vi "Configure SPI Source.vi"(7 "Source Type (0: Clock Source)":i32(ring) items=["Clock Source", "Data Source", "Frame Source", "MISO Source", "MOSI Source"], 8 "error in (no error)":errorcluster, 9 "SPI Source (0: Channel 1)":i32(ring) items=["Channel 1", "Channel 2", "Channel 3", "Channel 4", "Function 1", "Function 2", "Function 3", "Function 4", "Memory 1", "Memory 2", "Memory 3", "Memory 4", "Digital 0", "Digital 1", "Digital 2", "Digital 3", "Digital 4", "Digital 5", "Digital 6", "Digital 7", "Digital 8", "Digital 9", "Digital 10", "Digital 11", "Digital 12", "Digital 13", "Digital 14", "Digital 15"], 10 "Channel (1: Serial Bus 1)":i32(ring)=1 items=["Serial Bus 1"=1, "Serial Bus 2"=2, "Serial Bus 3"=3, "Serial Bus 4"=4], 11 "VISA resource name":refnum<visa-resource-name>) -> (0 "error out":errorcluster, 3 "VISA resource name out":refnum<visa-resource-name>)   [LabVIEW 2020, in "Agilent 90000 Series.lvlib"]
doc: "Configures the source for SPI serial bus."
uses:
  Agilent 90000 Series.lvlib
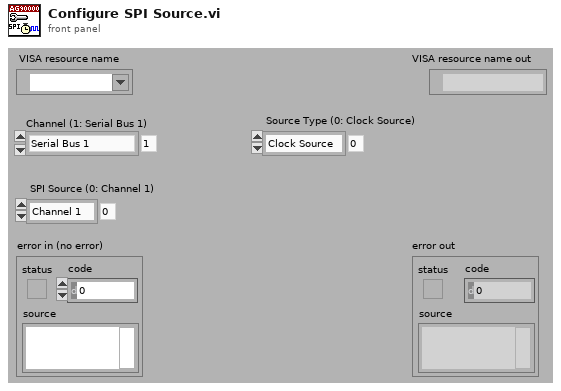
[diagram p1: front panel]
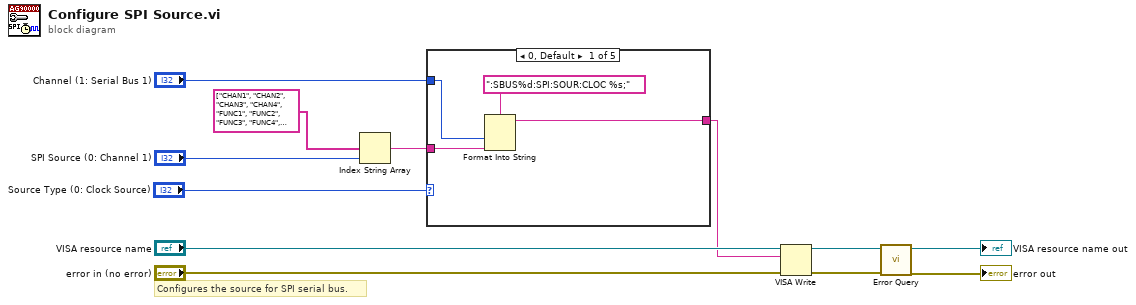
[diagram p0: block diagram]
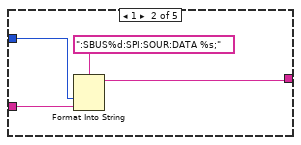
[diagram p2: hidden frame]
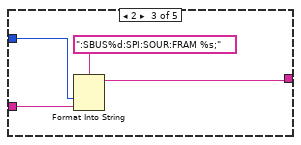
[diagram p3: hidden frame]
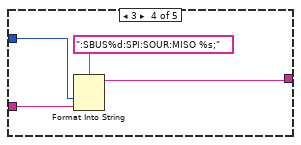
[diagram p4: hidden frame]
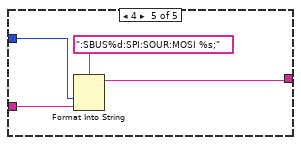
[diagram p5: hidden frame]
diagram:
  # "Configures the source for SPI serial bus."
  n1 = Index String Array(1:"SPI Source (0: Channel 1)", 2:string[] ["CHAN1", "CHAN2", "CHAN3", "CHAN4", "FUNC1", "FUNC2", "FUNC3", "FUNC4", "WMEM1", "WMEM2", "WMEM3", "WMEM4", "DIG0", "DIG1", "DIG2", "DIG3", "DIG4", "DIG5", "DIG6", "DIG7", "DIG8", "DIG9", "DIG10", "DIG11", "DIG12", "DIG13", "DIG14", "DIG15"]) -> (0:w2:string)  [unwired: 1 out]
  n2 = case shown="0, Default" "Source Type (0: Clock Source)" {
    tunnel: "Channel (1: Serial Bus 1)" -> [w16 w19 w23 w27 w31]
    tunnel: w2 -> [w15 w18 w22 w26 w30]
    tunnel: [w13 w17 w21 w25 w29] -> w1
    frame 0, Default {
      n3 = Format Into String(format string=":SBUS%d:SPI:SOUR:CLOC %s;", w16, w15) -> (resulting string=w13:string)  [unwired: 2 in, 1 out]
    }
    frame 1 {
      n4 = Format Into String(format string=":SBUS%d:SPI:SOUR:DATA %s;", w19, w18) -> (resulting string=w17:string)  [unwired: 2 in, 1 out]
    }
    frame 2 {
      n5 = Format Into String(format string=":SBUS%d:SPI:SOUR:FRAM %s;", w23, w22) -> (resulting string=w21:string)  [unwired: 2 in, 1 out]
    }
    frame 3 {
      n6 = Format Into String(format string=":SBUS%d:SPI:SOUR:MISO %s;", w27, w26) -> (resulting string=w25:string)  [unwired: 2 in, 1 out]
    }
    frame 4 {
      n7 = Format Into String(format string=":SBUS%d:SPI:SOUR:MOSI %s;", w31, w30) -> (resulting string=w29:string)  [unwired: 2 in, 1 out]
    }
  }
  n8 = VISA Write(VISA resource name="VISA resource name", write buffer=w1, error in (no error)="error in (no error)") -> (VISA resource name out=w10:refnum<visa-resource-name>, error out=w9:errorcluster)  [unwired: 1 out]
  n9 = call "Error Query.vi"("error in (no error)"=w9, "VISA resource name"=w10) -> ("error out"=→"error out":errorcluster, "VISA resource name out"=→"VISA resource name out":refnum<visa-resource-name>)  [unwired: 8 out]
